vi "AddBranchtoTree.vi"(9 "Child Node In":refnum<data-value>, 10 "Unique Node Name":string, 11 "Parent Node In":refnum<data-value>) -> (1 "Child Node Out (Cleared)":refnum<data-value>, 3 "Parent Node Out":refnum<data-value>)   [LabVIEW 2019]
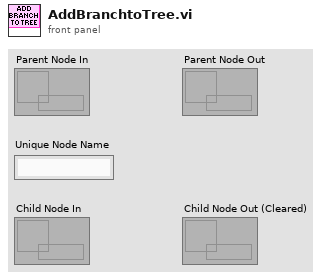
[diagram p1: front panel]
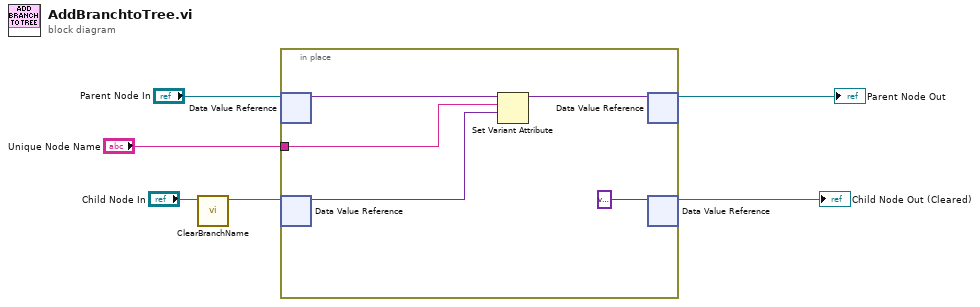
[diagram p0: block diagram]
diagram:
  n1 = call "ClearBranchName.vi"("Node In"="Child Node In") -> ("Node Out"=w1:refnum<data-value>)  [unwired: 9 in, 1 out]
  n2 = in-place {
    in-place-border: "Unique Node Name" -> [w8]
    n3 = in-place-dvr #1("Parent Node In") -> (w11:variant)  [unwired: 1 out]
    n4 = in-place-dvr #2(w1) -> (w7:variant)  [unwired: 1 out]
    n5 = Set Variant Attribute(Variant=w11, name=w8, value=w7) -> (Variant out=w10:variant)  [unwired: 1 in, 2 out]
    n6 = in-place-dvr #1(w10) -> (→"Parent Node Out":refnum<data-value>)  [unwired: 1 out]
    n7 = in-place-dvr #2(variant ("data value")) -> (→"Child Node Out (Cleared)":refnum<data-value>)  [unwired: 1 out]
  }
